vi "Pump Configure Speed.vi"(8 "error in (no error)":errorcluster, 10 "Message Data":variant, 11 "Data Cluster in":T1 {"Pump Info"."Direction" items=["CW", "CCW"]; "Pump Info"."Speed" format="%03.0f"}) -> (0 "error out":errorcluster, 3 "Data Cluster out":T1 {"Pump Info"."Direction" items=["CW", "CCW"]; "Pump Info"."Speed" format="%03.0f"})   [LabVIEW 2020, in "Pump.lvlib"]
uses:
  Pump.lvlib
  Pump Hardware Configuration.ctl
  support/Message Queue/Message Cluster.ctl
  support/HW Message Cluster.ctl
  support/Message Queue/Message Queue.lvlib
  <instrlib>/WM Pump/WM Pump.lvlib
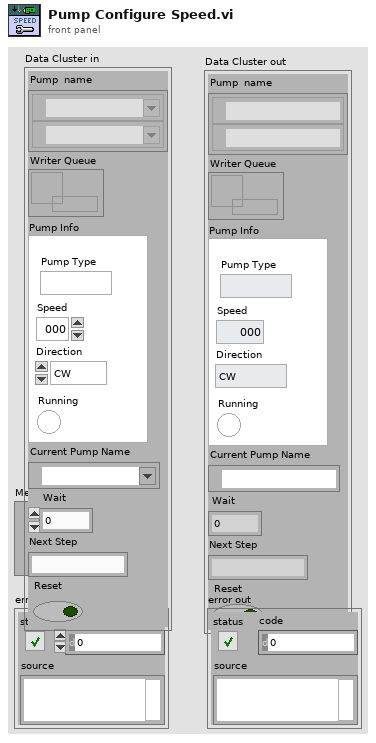
[diagram p1: front panel]
types:
  T1 = typedef "Pump.lvlib/Pump Hardware Configuration.ctl" = cluster{"Pump  name":refnum<visa-resource-name>[], "Writer Queue":refnum<queue>, "Pump Info":cluster{"Pump Type":string, "Speed":i32, "Direction":u16, "Running":bool}, "Current Pump Name":refnum<visa-resource-name>, "Wait":dbl, "Next Step":string, "Reset":bool}
  T2 = typedef "Message Queue.lvlib/HW Message Cluster.ctl" = cluster{"Writer Queue":refnum<queue>, "Writer Data":T3}
  T3 = typedef "Message Queue.lvlib/Message Cluster.ctl" = cluster{"Message":string, "Message Data":variant}
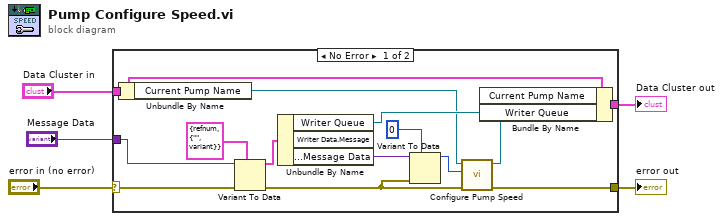
[diagram p0: block diagram]
diagram:
  n1 = case shown="No Error" "error in (no error)" {
    selector: "error in (no error)" -> [w16 w20]
    tunnel: "Message Data" -> [w15 _]
    tunnel: [w19 w21] -> w4
    tunnel: "Data Cluster in" -> [w18 w21]
    tunnel: [w6 w20] -> w2
    frame No Error {
      n2 = Unbundle By Name(w18) -> ("Current Pump Name"=w11:refnum<visa-resource-name>)
      n3 = Variant To Data(error in=w16, type=T2 {"Writer Queue"=refnum, "Writer Data"={"Message"="", "Message Data"=variant}}, Variant=w15) -> (data=w17:T2, error out=w10:errorcluster)
      n4 = Unbundle By Name(w17) -> ("Writer Queue"=w14:refnum<queue>, "Writer Data.Message Data"=w13:variant)  [unwired: 1 out]
      n5 = Variant To Data(error in=w10, type=0 ("Speed"), Variant=w13) -> (data=w8:i32)  [unwired: 1 out]
      n6 = call <instrlib>:"Configure Pump Speed.vi"("error in (no error)"=w10, "Speed"=w8, "VISA resource name"=w11) -> ("error out"=w6:errorcluster, "VISA resource name out"=w7:refnum<visa-resource-name>)  [unwired: 7 in]
      n7 = Bundle By Name(cluster=w18, "Current Pump Name"=w7, "Writer Queue"=w14) -> (w19:T1)
    }
    frame Error {
    }
  }
  "Data Cluster out" <- w4
  "error out" <- w2
